vi "OPC Connection Inspect.vi"() -> ()   [LabVIEW 2017]
uses:
  Global System.vi
panel:
  in  "G-PLC心跳":bool
  out "G-PC心跳":bool
  out "连接建立中":bool
  out "flag":bool
  out "数值":dbl
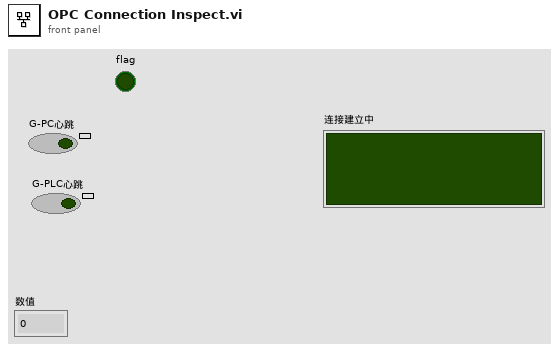
[diagram p1: front panel]
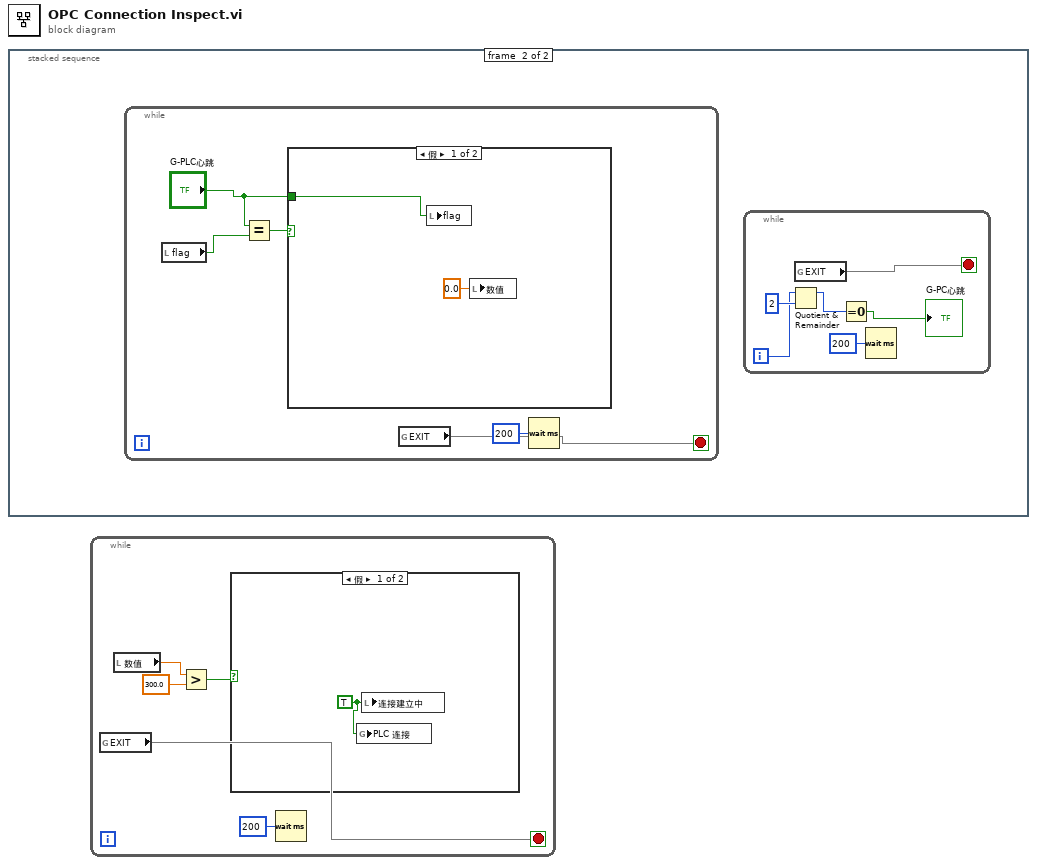
[diagram p0: block diagram]
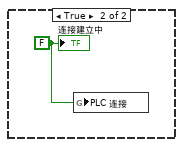
[diagram p2: hidden frame]
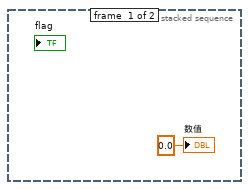
[diagram p3: hidden frame]
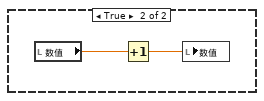
[diagram p4: hidden frame]
diagram:
  n1 = stacked-sequence {
    frame #0 {
      "数值" <- 0.0 ("数值")
    }
    frame #1 {
      n2 = while {
        stop <- w8 stop-if-true
        n3 = local read "flag"() -> (w12:bool)
        n4 = Equal?(x="G-PLC心跳", y=w12) -> (x = y?=w11:bool)
        n5 = case shown="假" w11 {
          tunnel: "G-PLC心跳" -> [w13 _]
          frame False {
            n6 = local write "flag"(w13) -> ()
            n7 = local write "数值"(0.0 ("数值")) -> ()
          }
          frame True {
            n8 = local read "数值"() -> (w16:dbl)
            n9 = Increment(x=w16) -> (x+1=w15:dbl)
            n10 = local write "数值"(w15) -> ()
          }
        }
        n11 = global read "Global System.vi" "EXIT"() -> (w8)
        n12 = Wait (ms)(milliseconds to wait=u32 200 ("等待时间（毫秒）")) -> ()  [unwired: 1 out]
      }
      n13 = while {
        i -> [w5]
        stop <- w2 stop-if-true
        n14 = Quotient & Remainder(x=w5, y=2) -> (x-y*floor(x/y)=w7:i32)  [unwired: 1 out]
        n15 = global read "Global System.vi" "EXIT"() -> (w2)
        n16 = Equal To 0?(x=w7) -> (x = 0?=→"G-PC心跳":bool)
        n17 = Wait (ms)(milliseconds to wait=u32 200 ("等待时间（毫秒）")) -> ()  [unwired: 1 out]
      }
    }
  }
  n18 = while {
    stop <- w17 stop-if-true
    n19 = global read "Global System.vi" "EXIT"() -> (w17)
    n20 = local read "数值"() -> (w20:dbl)
    n21 = Greater?(x=w20, y=300.0) -> (0:w21:bool)
    n22 = case shown="假" w21 {
      frame False {
        w22 = TRUE ("连接建立中")
        n23 = global write "Global System.vi" "PLC 连接"(w22) -> ()
        n24 = local write "连接建立中"(w22) -> ()
      }
      frame True {
        w23 = FALSE ("连接建立中")
        n25 = global write "Global System.vi" "PLC 连接"(w23) -> ()
        "连接建立中" <- w23
      }
    }
    n26 = Wait (ms)(milliseconds to wait=u32 200 ("等待时间（毫秒）")) -> ()  [unwired: 1 out]
  }
